vi "氨氮总磷总氮公式WR.vi"(6 "公式输入":cluster{"X^2":dbl, "X":dbl, "b":dbl}, 7 "STEP":enum16{"open", "read", "write", "close"}(ring)=enum."read", 8 "error in (no error)":errorcluster caption="错误输入（无错误）", 9 "量程":enum16{"低量程", "高量程"}(ring), 10 "测量模式":enum16{"水样测量", "空白核查", "跨度核查", "标样核查", "加标回收"}(ring), 11 "测量参数":enum16{"氨氮", "总磷", "总氮"}(ring)) -> (0 "error out":errorcluster caption="错误输出", 3 "公式":cluster{"X^2":dbl, "X":dbl, "b":dbl})   [LabVIEW 2016]
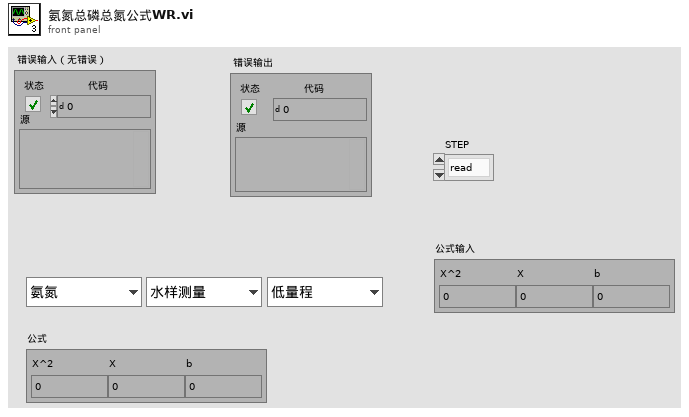
[diagram p1: front panel]
types:
  T1 = cluster{"FLOAT[0]":sgl, "FLOAT[1]":sgl, "FLOAT[2]":sgl}
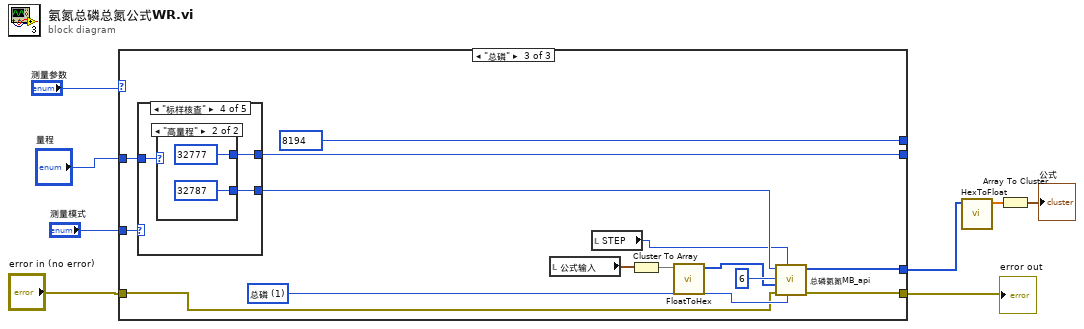
[diagram p0: block diagram]
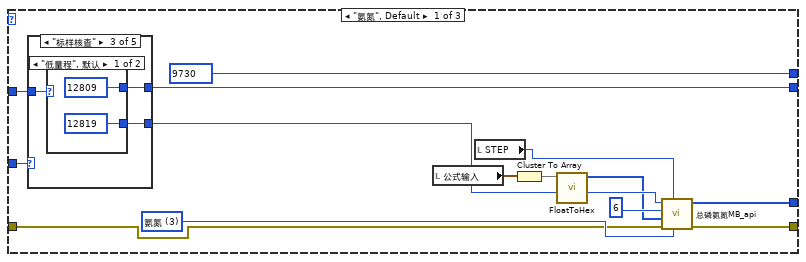
[diagram p2: hidden frame]
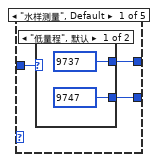
[diagram p3: hidden frame]
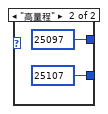
[diagram p4: hidden frame]
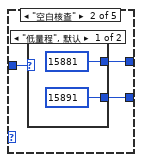
[diagram p5: hidden frame]
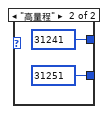
[diagram p6: hidden frame]
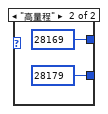
[diagram p7: hidden frame]
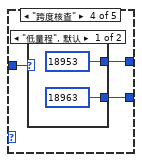
[diagram p8: hidden frame]
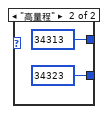
[diagram p9: hidden frame]
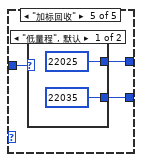
[diagram p10: hidden frame]
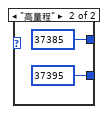
[diagram p11: hidden frame]
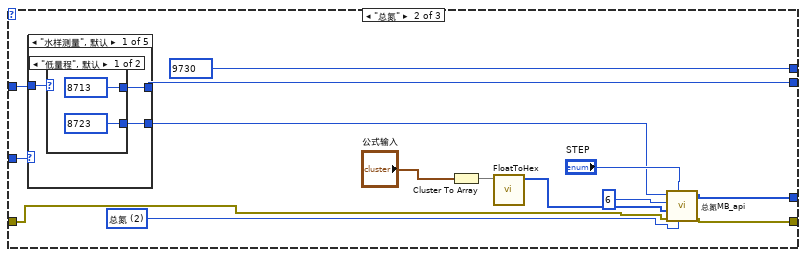
[diagram p12: hidden frame]
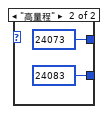
[diagram p13: hidden frame]
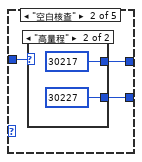
[diagram p14: hidden frame]
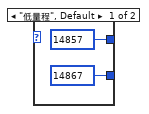
[diagram p15: hidden frame]
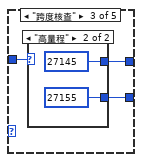
[diagram p16: hidden frame]
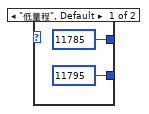
[diagram p17: hidden frame]
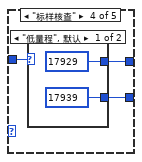
[diagram p18: hidden frame]
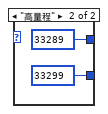
[diagram p19: hidden frame]
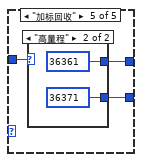
[diagram p20: hidden frame]
diagram:
  n1 = case shown="\"总磷\"" "测量参数" {
    tunnel: "测量模式" -> [w22 w70 w120]
    tunnel: "量程" -> [w21 w69 w119]
    tunnel: [w20 w68 w118] -> _
    tunnel: [u16 9730 ("starting address") u16 9730 ("starting address") u16 8194 ("starting address")] -> _
    tunnel: [w15 w63 w112] -> w2
    tunnel: "error in (no error)" -> [w14 w64 w111]
    tunnel: [w13 w61 w113] -> w1
    frame "氨氮", Default {
      w16 = u16 3 items=["总磷"=1, "总氮"=2, "氨氮"=3] ("站号")
      n2 = case shown="\"标样核查\"" w22 {
        tunnel: w21 -> [w25 w32 w39 w46 w53]
        tunnel: [w24 w31 w38 w45 w52] -> w17
        tunnel: [w23 w30 w37 w44 w51] -> w20
        frame "水样测量", Default {
          n3 = case shown="\"低量程\", 默认" w25 {
            tunnel: [u16 9747 ("starting address") u16 25107 ("starting address")] -> w24
            tunnel: [u16 9737 ("starting address") u16 25097 ("starting address")] -> w23
            frame "低量程", Default {
            }
            frame "高量程" {
            }
          }
        }
        frame "空白核查" {
          n4 = case shown="\"低量程\", 默认" w32 {
            tunnel: [u16 15891 ("starting address") u16 31251 ("starting address")] -> w31
            tunnel: [u16 15881 ("starting address") u16 31241 ("starting address")] -> w30
            frame "低量程", Default {
            }
            frame "高量程" {
            }
          }
        }
        frame "标样核查" {
          n5 = case shown="\"低量程\", 默认" w39 {
            tunnel: [u16 12819 ("starting address") u16 28179 ("starting address")] -> w38
            tunnel: [u16 12809 ("starting address") u16 28169 ("starting address")] -> w37
            frame "低量程", Default {
            }
            frame "高量程" {
            }
          }
        }
        frame "跨度核查" {
          n6 = case shown="\"低量程\", 默认" w46 {
            tunnel: [u16 18963 ("starting address") u16 34323 ("starting address")] -> w45
            tunnel: [u16 18953 ("starting address") u16 34313 ("starting address")] -> w44
            frame "低量程", Default {
            }
            frame "高量程" {
            }
          }
        }
        frame "加标回收" {
          n7 = case shown="\"低量程\", 默认" w53 {
            tunnel: [u16 22035 ("starting address") u16 37395 ("starting address")] -> w52
            tunnel: [u16 22025 ("starting address") u16 37385 ("starting address")] -> w51
            frame "低量程", Default {
            }
            frame "高量程" {
            }
          }
        }
      }
      n8 = local read "公式输入"() -> (w12:cluster{"X^2":dbl, "X":dbl, "b":dbl})
      n9 = local read "STEP"() -> (w10:enum16{"open", "read", "write", "close"})
      n10 = Cluster To Array(cluster=w12) -> (array=w11:dbl[])
      n11 = call "FloatToHex.vi"("浮点数"=w11) -> ("DCBA整形输出"=w9:u16[])  [unwired: 10 in]
      n12 = call "总磷氨氮MB_api.vi"("Slave ID"=w16, "STEP"=w10, "Error in"=w14, "values"=w9, "quantity"=u16 6, "starting address"=w17) -> ("error out"=w15:errorcluster, "Registers"=w13:u16[])  [unwired: 3 in, 1 out]
    }
    frame "总氮" {
      w62 = u16 2 items=["总磷"=1, "总氮"=2, "氨氮"=3] ("站号")
      n13 = case shown="\"水样测量\", 默认" w70 {
        tunnel: w69 -> [w74 w81 w88 w95 w102]
        tunnel: [w73 w80 w87 w94 w101] -> w66
        tunnel: [w72 w79 w86 w93 w100] -> w68
        frame "水样测量", Default {
          n14 = case shown="\"低量程\", 默认" w74 {
            tunnel: [u16 8723 ("starting address") u16 24083 ("starting address")] -> w73
            tunnel: [u16 8713 ("starting address") u16 24073 ("starting address")] -> w72
            frame "低量程", Default {
            }
            frame "高量程" {
            }
          }
        }
        frame "空白核查" {
          n15 = case shown="\"高量程\"" w81 {
            tunnel: [u16 14867 ("starting address") u16 30227 ("starting address")] -> w80
            tunnel: [u16 14857 ("starting address") u16 30217 ("starting address")] -> w79
            frame "低量程", Default {
            }
            frame "高量程" {
            }
          }
        }
        frame "跨度核查" {
          n16 = case shown="\"高量程\"" w88 {
            tunnel: [u16 11795 ("starting address") u16 27155 ("starting address")] -> w87
            tunnel: [u16 11785 ("starting address") u16 27145 ("starting address")] -> w86
            frame "低量程", Default {
            }
            frame "高量程" {
            }
          }
        }
        frame "标样核查" {
          n17 = case shown="\"低量程\", 默认" w95 {
            tunnel: [u16 17939 ("starting address") u16 33299 ("starting address")] -> w94
            tunnel: [u16 17929 ("starting address") u16 33289 ("starting address")] -> w93
            frame "低量程", Default {
            }
            frame "高量程" {
            }
          }
        }
        frame "加标回收" {
          n18 = case shown="\"高量程\"" w102 {
            tunnel: [u16 21011 ("starting address") u16 36371 ("starting address")] -> w101
            tunnel: [u16 21001 ("starting address") u16 36361 ("starting address")] -> w100
            frame "低量程", Default {
            }
            frame "高量程" {
            }
          }
        }
      }
      n19 = Cluster To Array(cluster="公式输入") -> (array=w59:dbl[])
      n20 = call "FloatToHex.vi"("浮点数"=w59) -> ("DCBA整形输出"=w58:u16[])  [unwired: 10 in]
      n21 = call "总氮MB_api.vi"("Slave ID"=w62, "STEP"="STEP", "Error in"=w64, "values"=w58, "quantity"=u16 6, "starting address"=w66) -> ("error out"=w63:errorcluster, "Registers"=w61:u16[])  [unwired: 3 in, 1 out]
    }
    frame "总磷" {
      w115 = u16 1 items=["总磷"=1, "总氮"=2, "氨氮"=3] ("站号")
      n22 = case shown="\"标样核查\"" w120 {
        tunnel: w119 -> [w123 w130 w137 w144 w151]
        tunnel: [w122 w129 w136 w143 w150] -> w114
        tunnel: [w121 w128 w135 w142 w149] -> w118
        frame "水样测量", Default {
          n23 = case shown="\"低量程\", 默认" w123 {
            tunnel: [u16 8211 ("starting address") u16 23571 ("starting address")] -> w122
            tunnel: [u16 8201 ("starting address") u16 23561 ("starting address")] -> w121
            frame "低量程", Default {
            }
            frame "高量程" {
            }
          }
        }
        frame "空白核查" {
          n24 = case shown="\"低量程\", 默认" w130 {
            tunnel: [u16 14355 ("starting address") u16 29715 ("starting address")] -> w129
            tunnel: [u16 14345 ("starting address") u16 29705 ("starting address")] -> w128
            frame "低量程", Default {
            }
            frame "高量程" {
            }
          }
        }
        frame "跨度核查" {
          n25 = case shown="\"高量程\"" w137 {
            tunnel: [u16 11283 ("starting address") u16 26643 ("starting address")] -> w136
            tunnel: [u16 11273 ("starting address") u16 26633 ("starting address")] -> w135
            frame "低量程", Default {
            }
            frame "高量程" {
            }
          }
        }
        frame "标样核查" {
          n26 = case shown="\"高量程\"" w144 {
            tunnel: [u16 17427 ("starting address") u16 32787 ("starting address")] -> w143
            tunnel: [u16 17417 ("starting address") u16 32777 ("starting address")] -> w142
            frame "低量程", Default {
            }
            frame "高量程" {
            }
          }
        }
        frame "加标回收" {
          n27 = case shown="\"高量程\"" w151 {
            tunnel: [u16 20499 ("starting address") u16 35859 ("starting address")] -> w150
            tunnel: [u16 20489 ("starting address") u16 35849 ("starting address")] -> w149
            frame "低量程", Default {
            }
            frame "高量程" {
            }
          }
        }
      }
      n28 = local read "公式输入"() -> (w110:cluster{"X^2":dbl, "X":dbl, "b":dbl})
      n29 = local read "STEP"() -> (w108:enum16{"open", "read", "write", "close"})
      n30 = Cluster To Array(cluster=w110) -> (array=w109:dbl[])
      n31 = call "FloatToHex.vi"("浮点数"=w109) -> ("DCBA整形输出"=w107:u16[])  [unwired: 10 in]
      n32 = call "总磷氨氮MB_api.vi"("Slave ID"=w115, "STEP"=w108, "Error in"=w111, "values"=w107, "quantity"=u16 6, "starting address"=w114) -> ("error out"=w112:errorcluster, "Registers"=w113:u16[])  [unwired: 3 in, 1 out]
    }
  }
  "error out" <- w2
  n33 = call "HexToFloat.vi"("数组"=w1) -> ("FLOAT"=w5:sgl[])  [unwired: 10 in]
  n34 = Array To Cluster(array=w5) -> (cluster=→"公式":T1)
